vi "Read Columnname_Alais.vi"(8 "error in (no error)":errorcluster, 11 "SQLite in":refnum<class "SQLite.lvclass">) -> (0 "error out":errorcluster, 2 "Columnname_Alais":string[](array[string]), 3 "SQLite out":refnum<class "SQLite.lvclass">)   [LabVIEW 2017]
uses:
  SQLite.lvclass
  \\vmware-host\Shared Folders/D/Dev/NJAL/OP140/OP140_NJAL_valve_EOL_Test_20210806/Source_Public/DataBase/Top DB/TopDBClass.lvclass
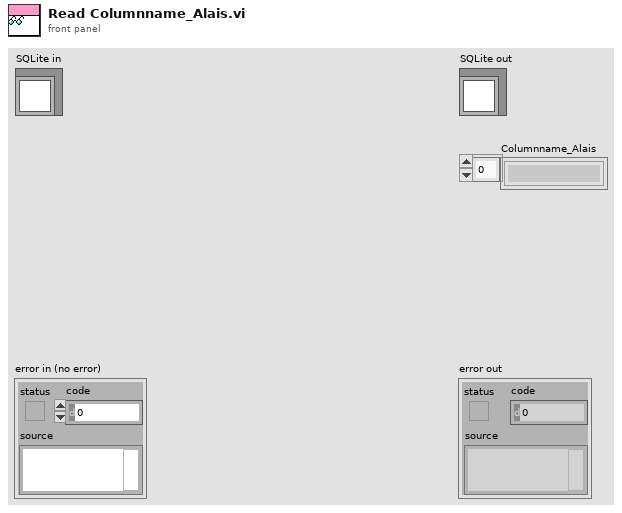
[diagram p1: front panel]
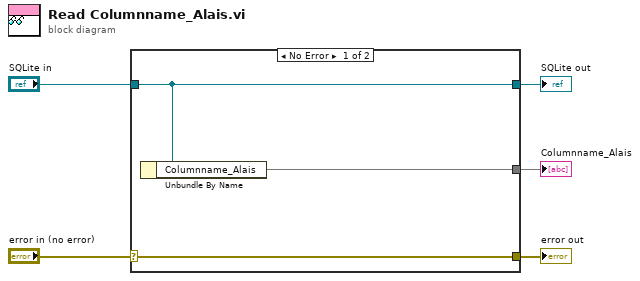
[diagram p0: block diagram]
diagram:
  n1 = case shown="No Error" "error in (no error)" {
    selector: "error in (no error)" -> [w8 w9]
    tunnel: [w8 w9] -> w4
    tunnel: [w7 w10] -> w2
    tunnel: "SQLite in" -> [w7 w10]
    tunnel: [w6 _] -> w1
    frame No Error {
      n2 = Unbundle By Name(w7) -> ("Columnname_Alais"=w6)
    }
    frame Error {
    }
  }
  "error out" <- w4
  "SQLite out" <- w2
  "Columnname_Alais" <- w1
